vi "Read Actors.vi"(8 "error in (no error)":errorcluster, 11 "CS++MessageMakerMain in":refnum<class "CS++MessageMakerMain.lvclass">) -> (0 "error out":errorcluster, 2 "Actors":refnum<class "CS++Actor.lvclass">[](array[class]), 3 "CS++MessageMakerMain out":refnum<class "CS++MessageMakerMain.lvclass">)   [LabVIEW 2016, in "CS++MessageMakerMain.lvlib" / "CS++MessageMakerMain.lvclass"]
uses:
  CS++MessageMakerMain.lvclass
  CSPP_Actor/CS++Actor.lvclass
  CS++MessageMakerMain.lvclass/CS++MessageMakerMain.ctl
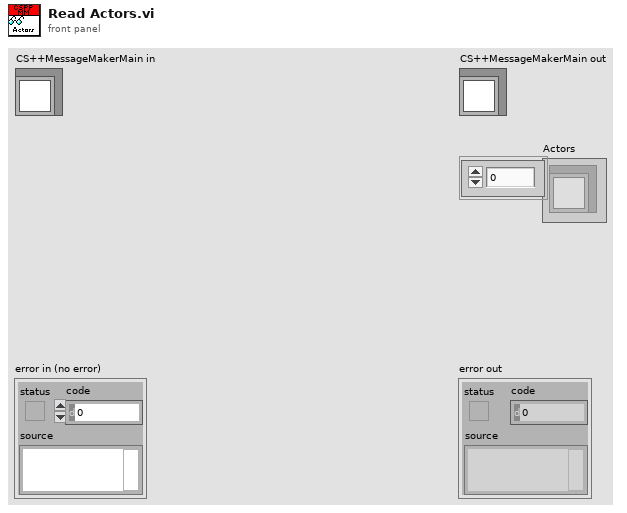
[diagram p1: front panel]
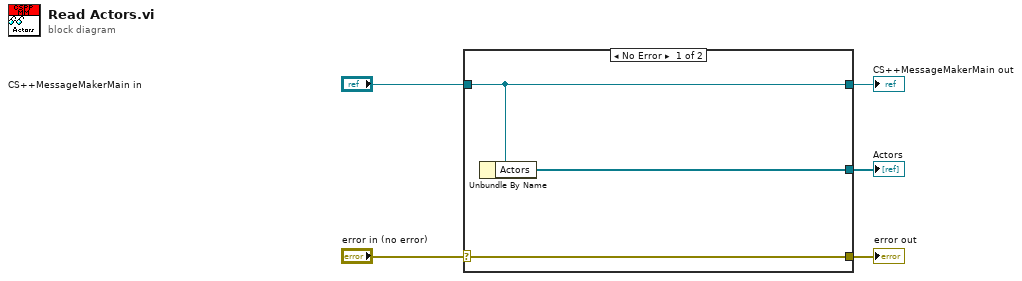
[diagram p0: block diagram]
diagram:
  n1 = case shown="No Error" "error in (no error)" {
    selector: "error in (no error)" -> [w8 w9]
    tunnel: [w8 w9] -> w4
    tunnel: [w7 w10] -> w2
    tunnel: "CS++MessageMakerMain in" -> [w7 w10]
    tunnel: [w6 _] -> w1
    frame No Error {
      n2 = Unbundle By Name(w7) -> ("Actors"=w6:refnum<class "CS++Actor.lvclass">[])
    }
    frame Error {
    }
  }
  "error out" <- w4
  "CS++MessageMakerMain out" <- w2
  "Actors" <- w1
